vi "SliceModel.vi"(11 "Z":dbl) -> (3 "Polys":T1[](array[typedef]))   [LabVIEW 2014]
uses:
  TypeDefs/Poly2DwSlope.ctl
  TypeDefs/Point2DwSlope.ctl
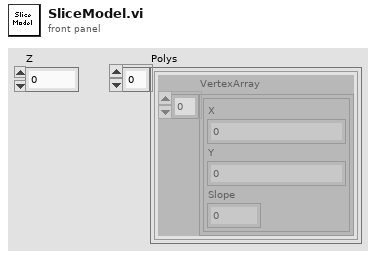
[diagram p1: front panel]
types:
  T1 = typedef "Poly2DwSlope.ctl" = cluster{"VertexArray":T2[]}
  T2 = typedef "Point2DwSlope.ctl" = cluster{"X":sgl, "Y":sgl, "Slope":dbl}
  T3 = typedef "TriangleFace.ctl" = cluster{"Normal":T4, "Vertex1":T4, "Vertex2":T4, "Vertex3":T4}
  T4 = typedef "Point3D.ctl" = cluster{"X":sgl, "Y":sgl, "Z":sgl}
  T5 = typedef "Line2D.ctl" = cluster{"Vertex1":T2, "Vertex2":T2, "Slope":dbl}
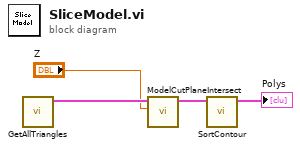
[diagram p0: block diagram]
diagram:
  n1 = call "GetAllTriangles.vi"() -> ("AllTriangles"=w3:T3[])  [unwired: 11 in]
  n2 = call "ModelCutPlaneIntersect.vi"("CuttingZ"="Z", "Triangles"=w3) -> ("LineArray"=w1:T5[])  [unwired: 8 in, 1 out]
  n3 = call "SortContour.vi"("LineArray"=w1) -> ("Polys"=→"Polys":T1[])  [unwired: 10 in]
